vi "Check Method Client Streaming.vi"(8 "error in (no error)":errorcluster, 11 "Method ref in":u64) -> (0 "error out":errorcluster, 2 "is Client Streaming":bool, 3 "Method ref out":u64)   [LabVIEW 2020, in "gRPC Scripting Tools.lvlib"]
uses:
  gRPC Scripting Tools.lvlib
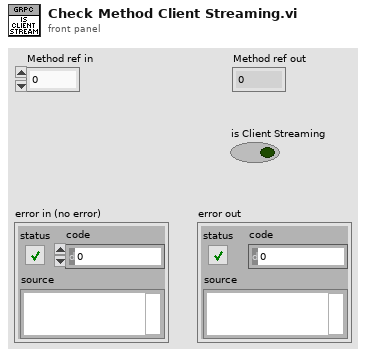
[diagram p1: front panel]
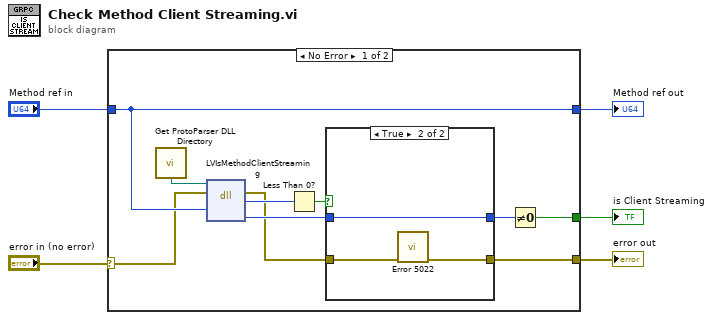
[diagram p0: block diagram]
diagram:
  n1 = case shown="No Error" "error in (no error)" {
    selector: "error in (no error)" -> [w12 w22]
    tunnel: "Method ref in" -> [w13 w21]
    tunnel: [w15 _] -> w4
    tunnel: [w13 w21] -> w3
    tunnel: [w6 w22] -> w1
    frame No Error {
      n2 = call "Get ProtoParser DLL Directory.vi"() -> ("Proto Parser Directory"=w14:path)
      n3 = dll-call lib="C:/Users/XEnderMD/Desktop/LV gRPC/labview source/gRPC Scripting Tools/Proto Parser API/dll/labview_grpc_generator.dll" fn="LVIsMethodClientStreaming"(path in=w14, error in=w12, "method"=w13) -> (error out=w7:errorcluster, "return type"=w11:i32, "clientStreaming"=w9:i32)  [unwired: 3 in, 1 out]
      n4 = Less Than 0?(x=w11) -> (x < 0?=w10:bool)
      n5 = case shown="True" w10 {
        tunnel: w9 -> [w17 w20]
        tunnel: [w17 w20] -> w8
        tunnel: w7 -> [w16 w19]
        tunnel: [w16 w18] -> w6
        frame False {
        }
        frame True {
          n6 = call "Error 5022.vi"("error in (no error)"=w19) -> ("error out"=w18:errorcluster)  [unwired: 10 in]
        }
      }
      n7 = Not Equal To 0?(x=w8) -> (x != 0?=w15:bool)
    }
    frame Error {
    }
  }
  "is Client Streaming" <- w4
  "Method ref out" <- w3
  "error out" <- w1
